vi "scrubUnicode.vi"(7 "replacement (-)":string="-", 10 "suspectStringIn":string) -> (0 "UnicodeReplaced?":bool, 2 "cleanStringOut":string)   [LabVIEW 2022 SP3]
panel:
  # "Replaces any characters with ASCII code >127 with Replacement Character(s).\nMulti-byte characters only trigger a single replacement"
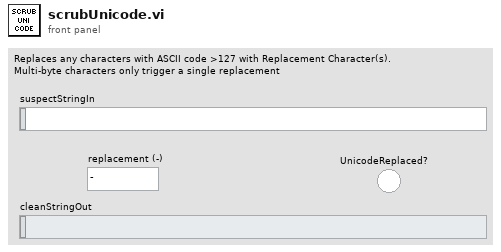
[diagram p1: front panel]
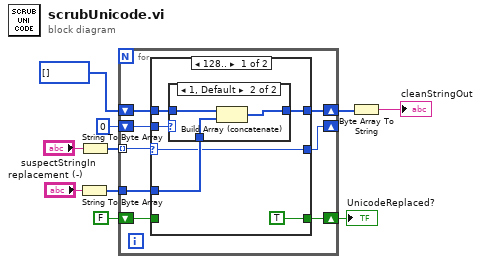
[diagram p0: block diagram]
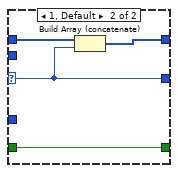
[diagram p3: hidden frame]
diagram:
  n1 = String To Byte Array(string="replacement (-)") -> (unsigned byte array=w6:u8[])
  n2 = String To Byte Array(string="suspectStringIn") -> (unsigned byte array=w9:u8[])
  n3 = for {
    tunnel: w9 -> [w18] mode=indexing
    tunnel: w6 -> [w17]
    shift-right: [w16] -> w5
    shift-left: u8[] [] -> [w15]
    shift-right: [w14] -> w2
    shift-left: FALSE -> [w13]
    shift-right: [w12] -> _
    shift-left: u8 0 -> [w11]
    n4 = case shown="128.." w18 {
      selector: w18 -> [w20 w29]
      tunnel: w17 -> [w23 _]
      tunnel: [w22 w32] -> w16
      tunnel: w15 -> [w24 w31]
      tunnel: [TRUE w30] -> w14
      tunnel: w13 -> [_ w30]
      tunnel: [w20 w29] -> w12
      tunnel: w11 -> [w19 _]
      frame 128.. {
        n5 = case shown="1, Default" w19 {
          tunnel: w24 -> [w25 w28]
          tunnel: w23 -> [_ w27]
          tunnel: [w25 w26] -> w22
          frame 128.. {
          }
          frame 1, Default {
            n6 = Build Array (concatenate)(w28, w27) -> (w26:u8[])
          }
        }
      }
      frame 1, Default {
        n7 = Build Array (concatenate)(w31, w29) -> (w32:u8[])
      }
    }
  }
  "UnicodeReplaced?" <- w2
  n8 = Byte Array To String(unsigned byte array=w5) -> (string=→"cleanStringOut":string)
